vi "dr_dtheta.vi"(1 "Wind Vector":cluster{"Wind R":dbl, "Wind Theta":dbl}, 3 "Boat Angle":dbl) -> (0 "dr/dt":dbl)   [LabVIEW 2011]
doc: "Given a wind vector and boat angle, returns the speed that the boat will approach the goal (assuming that the goal is at 0 degrees). This simply uses the estimated speed based on wind, and the cosine of the boat angle."
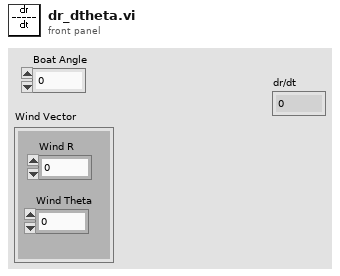
[diagram p1: front panel]
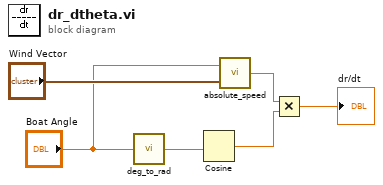
[diagram p0: block diagram]
diagram:
  n1 = call "deg_to_rad.vi"("Degrees"="Boat Angle") -> ("Radians"=w6:dbl)
  n2 = Cosine(x=w6) -> (cos(x)=w2:dbl)
  n3 = call "absolute_speed.vi"("Wind Vector"="Wind Vector", "Boat Angle"="Boat Angle") -> ("Velocity"=w4:dbl)
  n4 = Multiply(x=w4, y=w2) -> (x*y=→"dr/dt":dbl)
